vi "Main.vi"() -> ()   [LabVIEW 2017]
doc: "The myRIO Project template acquires acceleration data from the onboard accelerometer and displays the changes of acceleration values in a waveform chart."
uses:
  Main control.ctl
  Input Selection Control.ctl
panel:
  in  "Ground Switch":bool
  in  "Near tower":bool
  in  "Tower on End":bool
  in  "Rotation":bool
  in  "Reset/emergency Break":bool
  in  "Height":bool
  in  "Angle":bool
  in  "Length":bool
  in  "Next":bool
  # "selection buttons"
  # "Limit Switches"
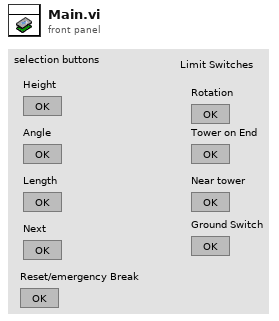
[diagram p1: front panel]
types:
  T1 = typedef "Main control.ctl" = enum16{"Initialize", "Main Menu", "Start Point", "End Point", "Move to Point"}
  T2 = typedef "Input Selection Control.ctl" = enum16{"Select Input", "Length", "Height", "Angle"}
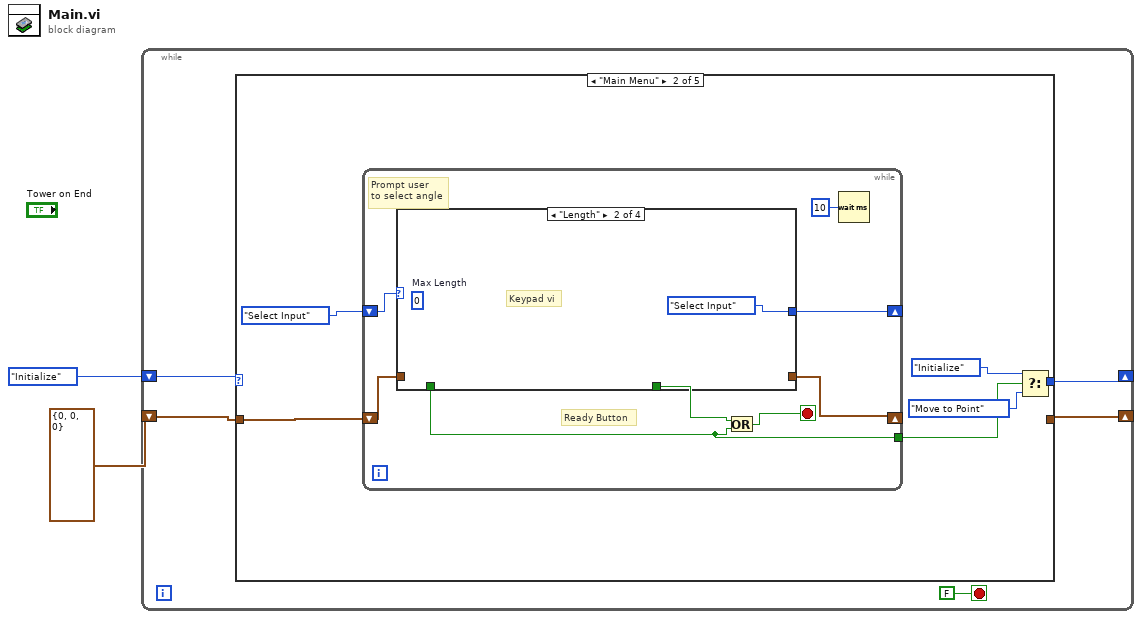
[diagram p0: block diagram]
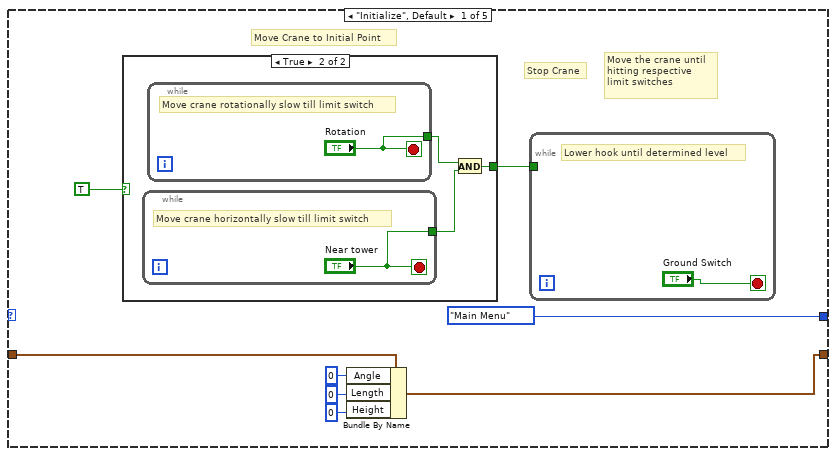
[diagram p2: hidden frame]
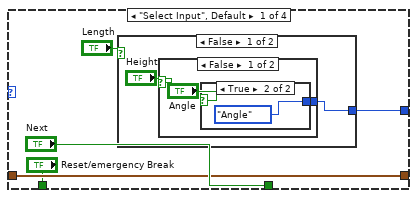
[diagram p4: hidden frame]
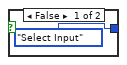
[diagram p5: hidden frame]
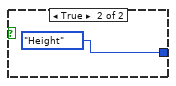
[diagram p6: hidden frame]
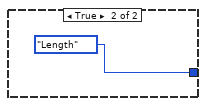
[diagram p7: hidden frame]
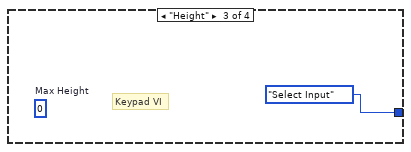
[diagram p8: hidden frame]
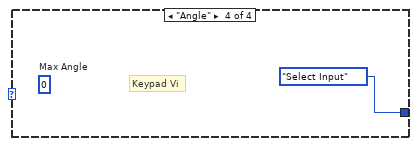
[diagram p9: hidden frame]
diagram:
  n1 = while {
    shift-right: [w6] -> _
    shift-left: Main_control."Initialize" -> [w7]
    shift-right: [w4] -> _
    shift-left: cluster{"Angle":i32, "Length":i32, "Height":i32} {"Angle"=0, "Length"=0, "Height"=0} -> [w5]
    stop <- FALSE stop-if-true
    n2 = case shown="\"Main Menu\"" w7 {
      tunnel: [Main_control."Main Menu" w27 _ _ _] -> w6
      tunnel: w5 -> [w10 w26 _ w52 _]
      tunnel: [w14 _ _ w52 _] -> w4
      frame "Initialize", Default {
        # "Move the crane until\nhitting respective \nlimit switches"
        # "Move Crane to Initial Point"
        # "Stop Crane"
        n3 = case shown="True" TRUE {
          tunnel: [_ w17] -> w8
          frame False {
          }
          frame True {
            n4 = while {
              tunnel: ["Near tower"] -> w18
              stop <- "Near tower" stop-if-true
              # "Move crane horizontally slow till limit switch"
            }
            n5 = while {
              tunnel: ["Rotation"] -> w19
              stop <- "Rotation" stop-if-true
              # "Move crane rotationally slow till limit switch"
            }
            n6 = And(x=w19, y=w18) -> (x .and. y?=w17:bool)
          }
        }
        n7 = Bundle By Name(cluster=w10, "Angle"=0, "Length"=0 ("Lenght"), "Height"=0) -> (w14:cluster{"Angle":i32, "Length":i32, "Height":i32})
        n8 = while {
          tunnel: w8 -> [_]
          stop <- "Ground Switch" stop-if-true
          # "Lower hook until determined level"
        }
      }
      frame "Main Menu" {
        n9 = while {
          shift-right: [w34] -> _
          shift-left: w26 -> [w35]
          tunnel: [w30] -> w25
          shift-right: [w28] -> _
          shift-left: Input_Selection_Control."Select Input" -> [w29]
          stop <- w31 stop-if-true
          # "Ready Button"
          # "Prompt user\nto select angle"
          n10 = case shown="\"Length\"" w29 {
            tunnel: ["Next" _ _ _] -> w32
            tunnel: w35 -> [w39 _ _ _]
            tunnel: [w39 _ _ _] -> w34
            tunnel: ["Reset/emergency Break" _ _ _] -> w30
            tunnel: [w36 Input_Selection_Control."Select Input" Input_Selection_Control."Select Input" Input_Selection_Control."Select Input"] -> w28
            frame "Select Input", Default {
              n11 = case shown="False" "Length" {
                tunnel: [w41 Input_Selection_Control."Length"] -> w36
                frame False {
                  n12 = case shown="False" "Height" {
                    tunnel: [w43 Input_Selection_Control."Height"] -> w41
                    frame False {
                      n13 = case shown="True" "Angle" {
                        tunnel: [Input_Selection_Control."Select Input" Input_Selection_Control."Angle"] -> w43
                        frame False {
                        }
                        frame True {
                        }
                      }
                    }
                    frame True {
                    }
                  }
                }
                frame True {
                }
              }
            }
            frame "Length" {
              (unwired) 0  # Max Length
              # "Keypad vi"
            }
            frame "Height" {
              (unwired) 0  # Max Height
              # "Keypad VI"
            }
            frame "Angle" {
              (unwired) 0  # Max Angle
              # "Keypad Vi"
            }
          }
          n14 = Or(x=w32, y=w30) -> (x .or. y?=w31:bool)
          n15 = Wait (ms)(milliseconds to wait=u32 10) -> ()  [unwired: 1 out]
        }
        n16 = Select(t=Main_control."Initialize", s=w25, f=Main_control."Move to Point") -> (s? t:f=w27:T1)
      }
      frame "End Point" {
      }
      frame "Move to Point" {
        # "Moves to input value point"
        n17 = while {
          stop <- _ stop-if-true
          # "Move to correct Height\nusing PID"
        }
        n18 = while {
          stop <- _ stop-if-true
          # "Move to correct rotation\nusing PID"
        }
        n19 = while {
          stop <- _ stop-if-true
          # "Move to correct length\nusing PID"
        }
      }
      frame "Start Point" {
      }
    }
  }
